vi "Report.vi"(6 "文件重命名":bool, 7 "文件名称":string, 8 "错误输入（无错误）":errorcluster, 11 "检测结果":bool[][](array[boolean])=[[TRUE]]) -> (0 "error out":errorcluster caption="错误输出", 3 "PRODUCT_VAULE":string)   [LabVIEW 2020]
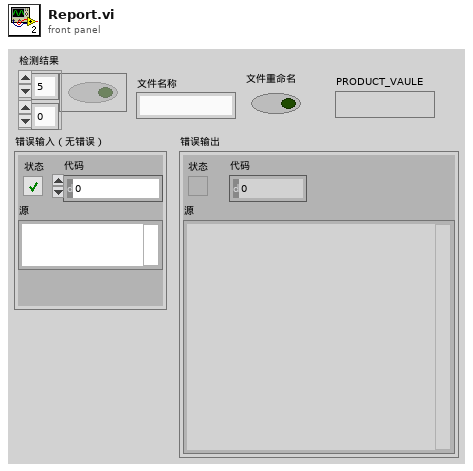
[diagram p1: front panel]
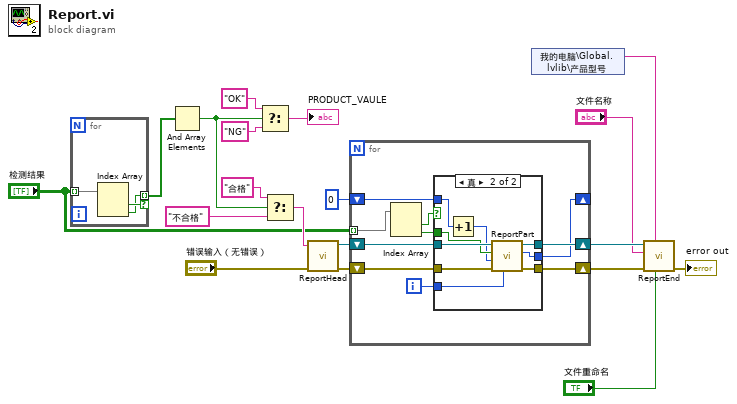
[diagram p0: block diagram]
diagram:
  n1 = for {
    tunnel: [w20] -> w4 mode=indexing if=w21
    tunnel: "检测结果" -> [w22] mode=indexing
    n2 = Index Array(array=w22) -> (element #1=w21:bool, element #2=w20:bool)  [unwired: 2 in]
  }
  n3 = And Array Elements(Boolean array=w4) -> (logical AND=w5:bool)
  n4 = Select(t="OK", s=w5, f="NG") -> (s? t:f=→"PRODUCT_VAULE":string)
  n5 = Select(t="合格", s=w5, f="不合格") -> (s? t:f=w10:string)
  n6 = call "ReportHead.vi"("error in (no error)"="错误输入（无错误）", "产品状态"=w10) -> ("error out"=w18:errorcluster, "report out"=w19:refnum<class "NI_report.lvclass">)  [unwired: 8 in]
  n7 = for {
    shift-right: [w30] -> w17
    shift-left: w19 -> [w32]
    shift-right: [w29] -> w16
    shift-left: w18 -> [w31]
    tunnel: "检测结果" -> [w25] mode=indexing
    shift-right: [w26] -> _
    shift-left: 0 ("索引OUT") -> [w27]
    i -> [w28]
    n8 = Index Array(array=w25) -> (element #1=w24:bool, element #2=w23:bool)  [unwired: 2 in]
    n9 = case shown="真" w24 {
      tunnel: w32 -> [w34 w42]
      tunnel: w31 -> [w35 w43]
      tunnel: [w34 w40] -> w30
      tunnel: [w35 w38] -> w29
      tunnel: w28 -> [_ w44]
      tunnel: w23 -> [_ w37]
      tunnel: w27 -> [w33 w41]
      tunnel: [w33 w39] -> w26
      frame False {
      }
      frame True {
        n10 = Increment(x=w41) -> (x+1=w36:i32)
        n11 = call "ReportPart.vi"("试验项目"=w44, "error in"=w43, "索引IN"=w36, "合格"=w37, "report in"=w42) -> ("error out 2"=w38:errorcluster, "索引OUT"=w39:i32, "report out"=w40:refnum<class "NI_report.lvclass">)  [unwired: 4 in]
      }
    }
  }
  n12 = shared-variable "我的电脑\\Global.lvlib\\产品型号"() -> (w1:string)  [unwired: 1 in, 1 out]
  n13 = call "ReportEnd.vi"("文件重命名"="文件重命名", "产品型号"=w1, "error in (no error)"=w16, "文件名称"="文件名称", "report in"=w17) -> ("error out"=→"error out":errorcluster)  [unwired: 6 in]
